vi "test_Add Array Existing Ch. Name .vi"(8 "error in (no error)":errorcluster, 11 "TestCase in":refnum<class "Instrument Addon Scripting API Channels Unit Tests.lvclass">) -> (0 "error out":errorcluster, 3 "TestCase out":refnum<class "Instrument Addon Scripting API Channels Unit Tests.lvclass">)   [LabVIEW 2018, in "Instrument Addon Scripting API Channels Unit Tests.lvclass"]
uses:
  Instrument Addon Scripting API Channels Unit Tests.lvclass
  APIs/Scripting API/TypeDefs/Array Enumerated List Settings.ctl
  APIs/Scripting API/TypeDefs/Array Element.ctl
  Addon/Addon Shared/SubVIs/Constants.vi
  <vilib>/NI/NI VeriStand Advanced SysDef API/_SubVIs/SysDef.Search.GUID.vi
  APIs/Scripting API/Channels/Create Data Channel - Array - Enumerated List.vi
  <vilib>/NI/NI VeriStand Advanced SysDef API/_SubVIs/SysDef.Search.GUIDs.vi
  <vilib>/addons/_JKI Toolkits/VI Tester/TestCase.llb/TestCase.lvclass
  Instrument Addon Scripting API Test Assets/Instrument Addon Scripting API Test Assets.lvclass
  <vilib>/NI/NI VeriStand Advanced SysDef API/SysDef API/Advanced System Definition.lvlib
  Addon/Addon Shared/Instrument Addon Shared.lvlib
  APIs/Scripting API/Instrument Addon Scripting API.lvlib
  C:/Program Files (x86)/National Instruments/LabVIEW 2018/vi.lib/addons/_JKI Toolkits/VI Tester/TestCase.llb/TestCase.lvclass
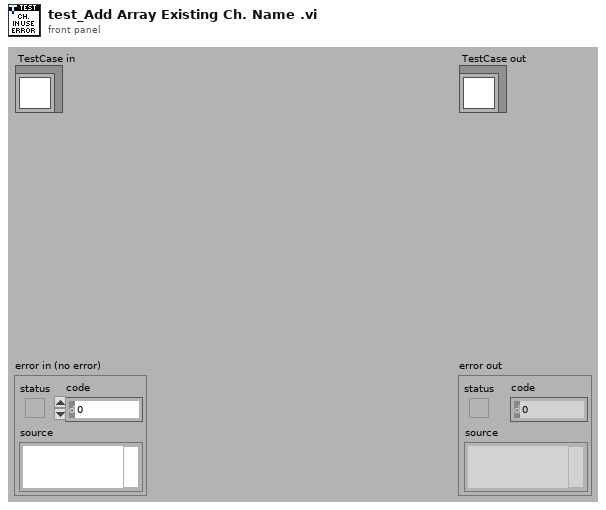
[diagram p1: front panel]
types:
  T1 = typedef "Instrument Addon Scripting API.lvlib/Array Enumerated List Settings.ctl" = cluster{"Elements":T2[], "Enumerated List":string[], "Delimiter":string}
  T2 = typedef "Instrument Addon Scripting API.lvlib/Array Element.ctl" = cluster{"Name":string, "Default Value":dbl, "Units":string}
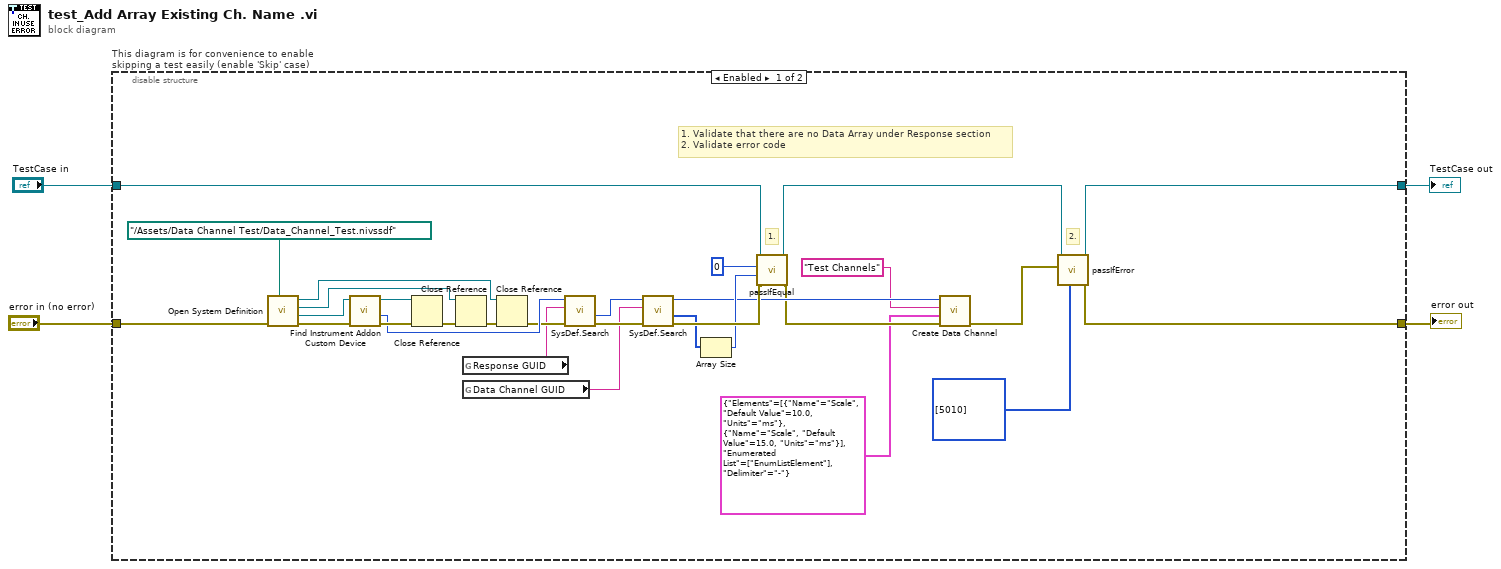
[diagram p0: block diagram]
diagram:
  n1 = disable-structure "This diagram is for convenience to enable skipping a test easily (enable 'Skip' case)" shown="Enabled" {
    disable-tunnel: "TestCase in" -> [w18 w38]
    disable-tunnel: [w6 w36] -> w1
    disable-tunnel: [w7 w37] -> w3
    disable-tunnel: "error in (no error)" -> [w25 w35]
    frame Enabled {
      # "2."
      # "1. Validate that there are no Data Array under Response section\n2. Validate error code"
      # "1."
      n2 = call "Open System Definition.vi"("error in (no error)"=w25, "System Definition File"=path "../Assets/Data Channel Test/Data_Channel_Test.nivssdf") -> ("error out"=w34:errorcluster, "Target Refnum"=w33:refnum<k24>, "Root Refnum"=w29:refnum<k24>, "System Definition Refnum"=w30:refnum<k24>)  [unwired: 6 in]
      n3 = call "Find Instrument Addon Custom Device.vi"("error in"=w34, "target in"=w33) -> ("error out"=w26:errorcluster, "NodeID"=w24:u64, "target out"=w27:refnum<k24>)  [unwired: 7 in]
      n4 = Close Reference(reference=w27, error in (no error)=w26) -> (error out=w28:errorcluster)
      n5 = Close Reference(reference=w29, error in (no error)=w28) -> (error out=w31:errorcluster)
      n6 = global read "Constants.vi" "Response GUID"() -> (w22:string)
      n7 = global read "Constants.vi" "Data Channel GUID"() -> (w19:string)
      n8 = Close Reference(reference=w30, error in (no error)=w31) -> (error out=w23:errorcluster)
      n9 = call-poly <vilib>:"SysDef.Search.vi"("error in (no error)"=w23, "GUID"=w22, "nodeID"=w24) -> ("error out"=w20:errorcluster, "Value out"=w21:u64)  [unwired: 5 in, 2 out]
      n10 = call-poly <vilib>:"SysDef.Search.vi"("error in (no error)"=w20, "GUID"=w19, "nodeID"=w21) -> ("error out"=w16:errorcluster, "Values Out"=w15:u64[], "nodeID out"=w12:u64)  [unwired: 5 in, 1 out]
      n11 = Array Size(array=w15) -> (size(s)=w14:i32)
      n12 = call-dynamic "passIfEqual.vi"("error in (no error)"=w16, "y"=w14, "x"=0 ("size(s)"), "TestCase in"=w18) -> ("error out"=w11:errorcluster, "TestCase out"=w17:refnum<class "Instrument Addon Scripting API Channels Unit Tests.lvclass">)  [unwired: 6 in]
      n13 = call-poly "Create Data Channel.vi"("Error In"=w11, "Settings"=T1 {"Elements"=[{"Name"="Scale", "Default Value"=10.0, "Units"="ms"}, {"Name"="Scale", "Default Value"=15.0, "Units"="ms"}], "Enumerated List"=["EnumListElement"], "Delimiter"="-"}, "Name"="Test Channels", "Message Refnum In"=w12) -> ("Error Out"=w5:errorcluster)  [unwired: 5 in, 2 out]
      n14 = call-dynamic "passIfError.vi"("passing error codes (default = any error code)"=i32[] [5010], "error"=w5, "TestCase in"=w17) -> ("error out"=w7:errorcluster, "TestCase out"=w6:refnum<class "Instrument Addon Scripting API Channels Unit Tests.lvclass">)  [unwired: 7 in]
    }
    frame Disabled {
      # "skip test result while test is under development"
      n15 = call <vilib>:"skip.vi"("error in (no error)"=w35, "TestCase in"=w38) -> ("error out"=w37:errorcluster, "TestCase out"=w36:refnum<class "Instrument Addon Scripting API Channels Unit Tests.lvclass">)  [unwired: 8 in]
    }
  }
  "error out" <- w3
  "TestCase out" <- w1
